vi "ShouldIncludeIfExternal.vi"(8 "error in (no error)":errorcluster, 9 "Current item":refnum<class "ILabVIEWItem.lvclass">, 10 "Include external?":bool, 11 "CLabVIEWContainer in":refnum<class "CLabVIEWContainer.lvclass">) -> (0 "error out":errorcluster, 1 "Include?":bool, 3 "CLabVIEWContainer out":refnum<class "CLabVIEWContainer.lvclass">)   [LabVIEW 2020, in "LabVIEWContainers.lvlib" / "CLabVIEWContainer.lvclass"]
uses:
  CLabVIEWContainer.lvclass
  obj/Addons/LabVIEWObjectInterfaces.lvlibp/LabVIEWObjectInterfaces/ILabVIEWItem/ILabVIEWItem.lvclass
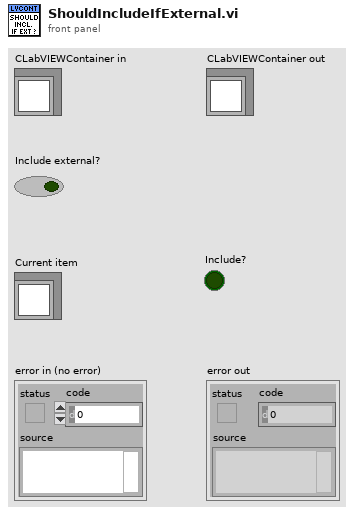
[diagram p1: front panel]
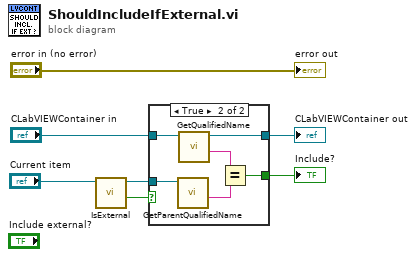
[diagram p0: block diagram]
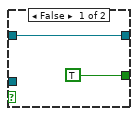
[diagram p2: hidden frame]
diagram:
  n1 = call-dynamic "IsExternal.vi"("ILabVIEWItem in"="Current item") -> ("Is external?"=w3:bool, "ILabVIEWItem out"=w2:refnum<class "ILabVIEWItem.lvclass">)  [unwired: 8 in, 1 out]
  n2 = case shown="True" w3 {
    tunnel: "CLabVIEWContainer in" -> [w8 w15]
    tunnel: [w8 w14] -> w5
    tunnel: w2 -> [_ w13]
    tunnel: [TRUE w10] -> w1
    frame False {
    }
    frame True {
      n3 = call-dynamic "GetParentQualifiedName.vi"("ILabVIEWItem in"=w13) -> ("Name"=w11:string)  [unwired: 8 in, 2 out]
      n4 = call-dynamic "GetQualifiedName.vi"("CLabVIEWItem in"=w15) -> ("Qualified name"=w12:string, "CLabVIEWItem out"=w14:refnum<class "CLabVIEWContainer.lvclass">)  [unwired: 8 in, 1 out]
      n5 = Equal?(x=w12, y=w11) -> (x = y?=w10:bool)
    }
  }
  "CLabVIEWContainer out" <- w5
  "Include?" <- w1
  "error out" <- "error in (no error)"
